vi "Update Bundle Definition Tree.vi"(6 "Bundle Filename":string, 7 "Reset Selection to Root? (T)":bool=TRUE, 8 "error in":errorcluster, 9 "Custom Actions File Names":string[](array[string]), 10 "Product List File Names":string[](array[string]), 11 "TreeControl in":refnum<vi>) -> (0 "error out":errorcluster, 3 "TreeControl out":refnum<vi>)   [LabVIEW 2020]
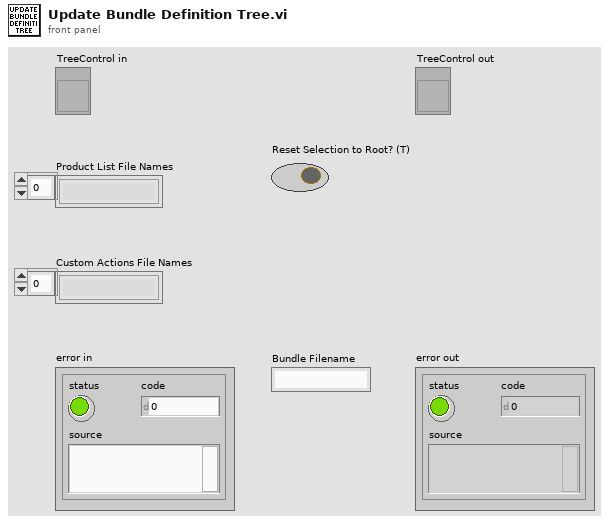
[diagram p1: front panel]
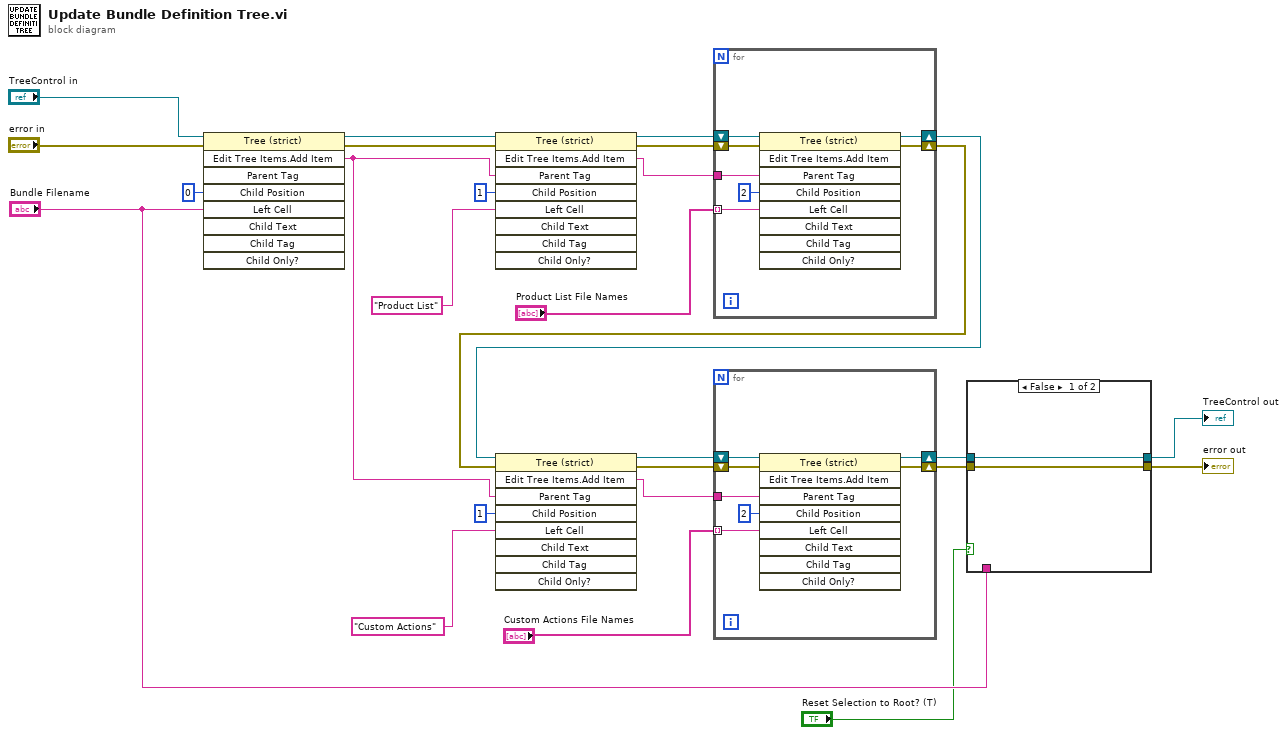
[diagram p0: block diagram]
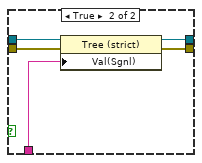
[diagram p2: hidden frame]
diagram:
  n1 = invoke class="Tree (strict)" method="Edit Tree Items.Add Item"(reference="TreeControl in", error in="error in", "Child Position"=0, "Left Cell"="Bundle Filename") -> (reference out=w21:refnum<vi>, error out=w24:errorcluster, "Edit Tree Items:Add Item"=w9:string)  [unwired: 5 in, 6 out]
  n2 = invoke class="Tree (strict)" method="Edit Tree Items.Add Item"(reference=w21, error in=w24, "Parent Tag"=w9, "Child Position"=1, "Left Cell"="Product List") -> (reference out=w18:refnum<vi>, error out=w22:errorcluster, "Edit Tree Items:Add Item"=w17:string)  [unwired: 4 in, 6 out]
  n3 = for {
    tunnel: w17 -> [w29]
    shift-right: [w32] -> w8
    shift-left: w22 -> [w33]
    shift-right: [w30] -> w10
    shift-left: w18 -> [w31]
    tunnel: "Product List File Names" -> [w27] mode=indexing
    n4 = invoke class="Tree (strict)" method="Edit Tree Items.Add Item"(reference=w31, error in=w33, "Parent Tag"=w29, "Child Position"=2, "Left Cell"=w27) -> (reference out=w30:refnum<vi>, error out=w32:errorcluster)  [unwired: 4 in, 7 out]
  }
  n5 = invoke class="Tree (strict)" method="Edit Tree Items.Add Item"(reference=w10, error in=w8, "Parent Tag"=w9, "Child Position"=1, "Left Cell"="Custom Actions") -> (reference out=w14:refnum<vi>, error out=w11:errorcluster, "Edit Tree Items:Add Item"=w15:string)  [unwired: 4 in, 6 out]
  n6 = for {
    tunnel: w15 -> [w36]
    shift-right: [w39] -> w6
    shift-left: w11 -> [w40]
    shift-right: [w37] -> w4
    shift-left: w14 -> [w38]
    tunnel: "Custom Actions File Names" -> [w34] mode=indexing
    n7 = invoke class="Tree (strict)" method="Edit Tree Items.Add Item"(reference=w38, error in=w40, "Parent Tag"=w36, "Child Position"=2, "Left Cell"=w34) -> (reference out=w37:refnum<vi>, error out=w39:errorcluster)  [unwired: 4 in, 7 out]
  }
  n8 = case shown="False" "Reset Selection to Root? (T)" {
    tunnel: w6 -> [w41 w47]
    tunnel: [w41 w46] -> w5
    tunnel: w4 -> [w42 w45]
    tunnel: "Bundle Filename" -> [_ w44]
    tunnel: [w42 w43] -> w2
    frame False {
    }
    frame True {
      n9 = property class="Tree (strict)"(reference=w45, error in=w47, "Val(Sgnl)"=w44) -> (reference out=w43:refnum<vi>, error out=w46:errorcluster)
    }
  }
  "TreeControl out" <- w2
  "error out" <- w5
